vi "ex2.vi"() -> ()   [LabVIEW 2019]
uses:
  <vilib>/express/express arith-compare/Formula/XNode/ExpressFormulaBlockNode.xnode
panel:
  in  "stop":bool
  out "Meter 3":dbl(knob) scale=0.0..10.0
  in  "U":dbl(knob) scale=0.0..10.0
  in  "R1":dbl(slide) scale=0.0..100.0
  out "Meter 2":dbl(knob) scale=0.0..10.0
  in  "U":dbl(knob) scale=0.0..10.0
  in  "R1":dbl(slide) scale=0.0..100.0
  in  "?":bool
  in  "?":bool
  in  "R1":dbl(slide) scale=0.0..100.0
  in  "U":dbl(knob) scale=0.0..10.0
  out "Meter":dbl(knob) scale=0.0..10.0
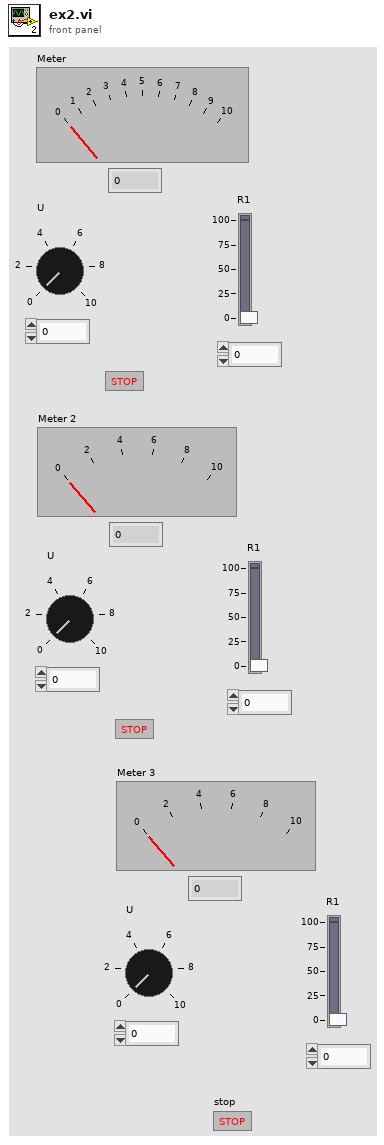
[diagram p1: front panel]
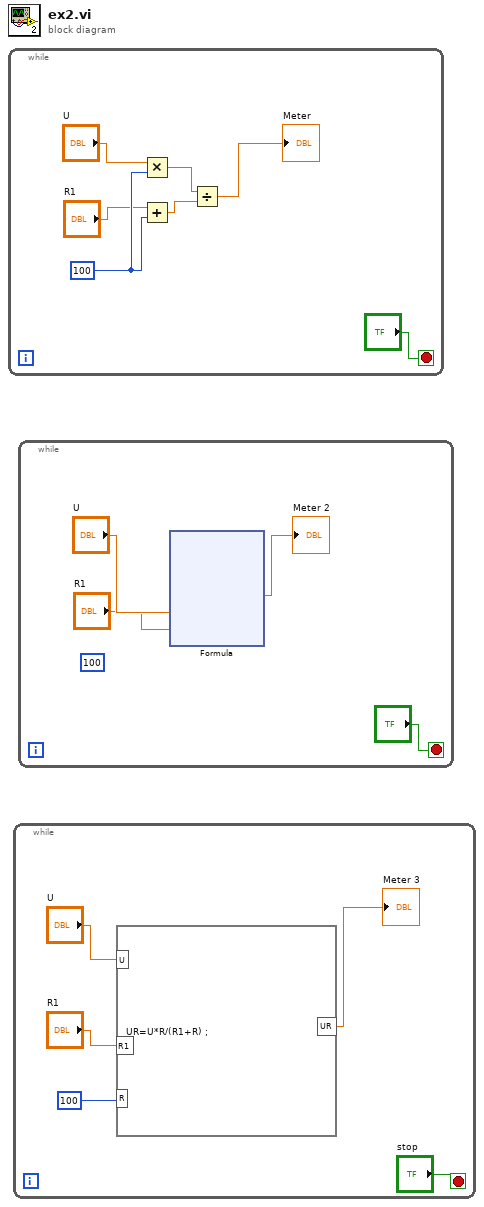
[diagram p0: block diagram]
diagram:
  n1 = while {
    stop <- "?" stop-if-true
    w5 = 100
    n2 = Multiply(x="U", y=w5) -> (x*y=w7:dbl)
    n3 = Add(x="R1", y=w5) -> (x+y=w6:dbl)
    n4 = Divide(x=w7, y=w6) -> (x/y=→"Meter":dbl)
  }
  n5 = while {
    stop <- "stop" stop-if-true
    n6 = formula code="UR=U*R/(R1+R) ;"("U"="U", "R"=100, "R1"="R1") -> ("UR"=→"Meter 3":dbl)
  }
  n7 = while {
    stop <- "?" stop-if-true
    (unwired) 100
    n8 = xnode "Formula"("U"="U", "R1"="R1") -> ("Result"=→"Meter 2":dbl)  [unwired: 1 in, 1 out]
  }
